vi "Constants.vi"() -> ()   [LabVIEW 2016, in "FPGA RM Test Client Shared.lvlib"]
doc: "Use this Global VI to access the GUIDs assigned to the page resources of the Custom Device."
uses:
  FPGA RM Test Client Shared.lvlib
panel:
  in  "Tab Control":enum32{"GUIDS", "Constants", "Properties"}(tab)
  in  "channel1":string="948f3141-7217-4176-9c74-7d56dae026b2"
  in  "channel0":string="307e6448-4571-40c0-8b53-8acd3873f7c7"
  in  "sub1":string="7807daf3-20a2-4b3b-b4a5-82fb83f35e86"
  in  "sub0":string="c45d75d1-215b-4c74-8a3e-0f64c6ad61f4"
  in  "FPGA RM Test Client":string="cb09ad27-7d84-4e9a-b6ff-fdadedd3d9b0"
  in  "Compiled.Settings":string="Compiled.Settings"
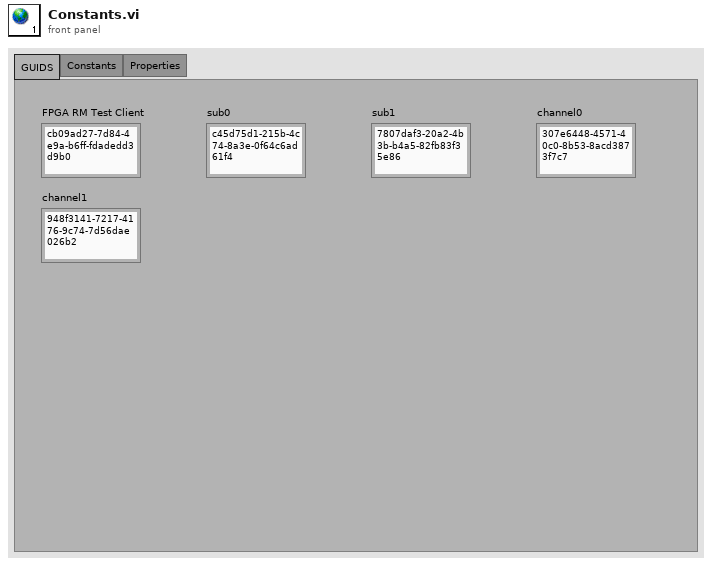
[diagram p1: front panel]
diagram:
